vi "Spectrometer.vi"() -> ()   [LabVIEW 2015]
uses:
  <vilib>/Utility/file.llb/Write Delimited Spreadsheet (DBL).vi
panel:
  out "x-y":dbl[](array[numeric])
  out "存储路径":path
  in  "确定按钮":bool
  in  "Stop Spectrum":bool
  out "Backlight Values":dbl[](array[numeric])
  in  "Save Backlight":bool
  in  "Enter the \nInetegration Time":i32=100
  out "Spectrum of the first Spectrometer":cluster{"Y":dbl[], "Y":dbl[]}[](graph)
  in  "Quit Program":bool
  in  "Spectrum Configure":bool
  out "Number of Spectrometers":i32
  # "ms"
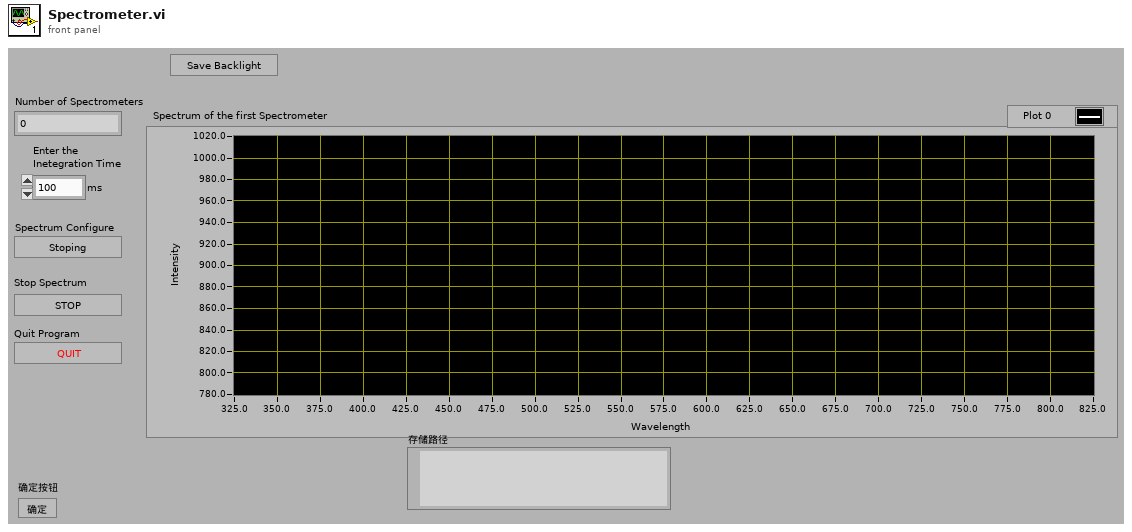
[diagram p1: front panel]
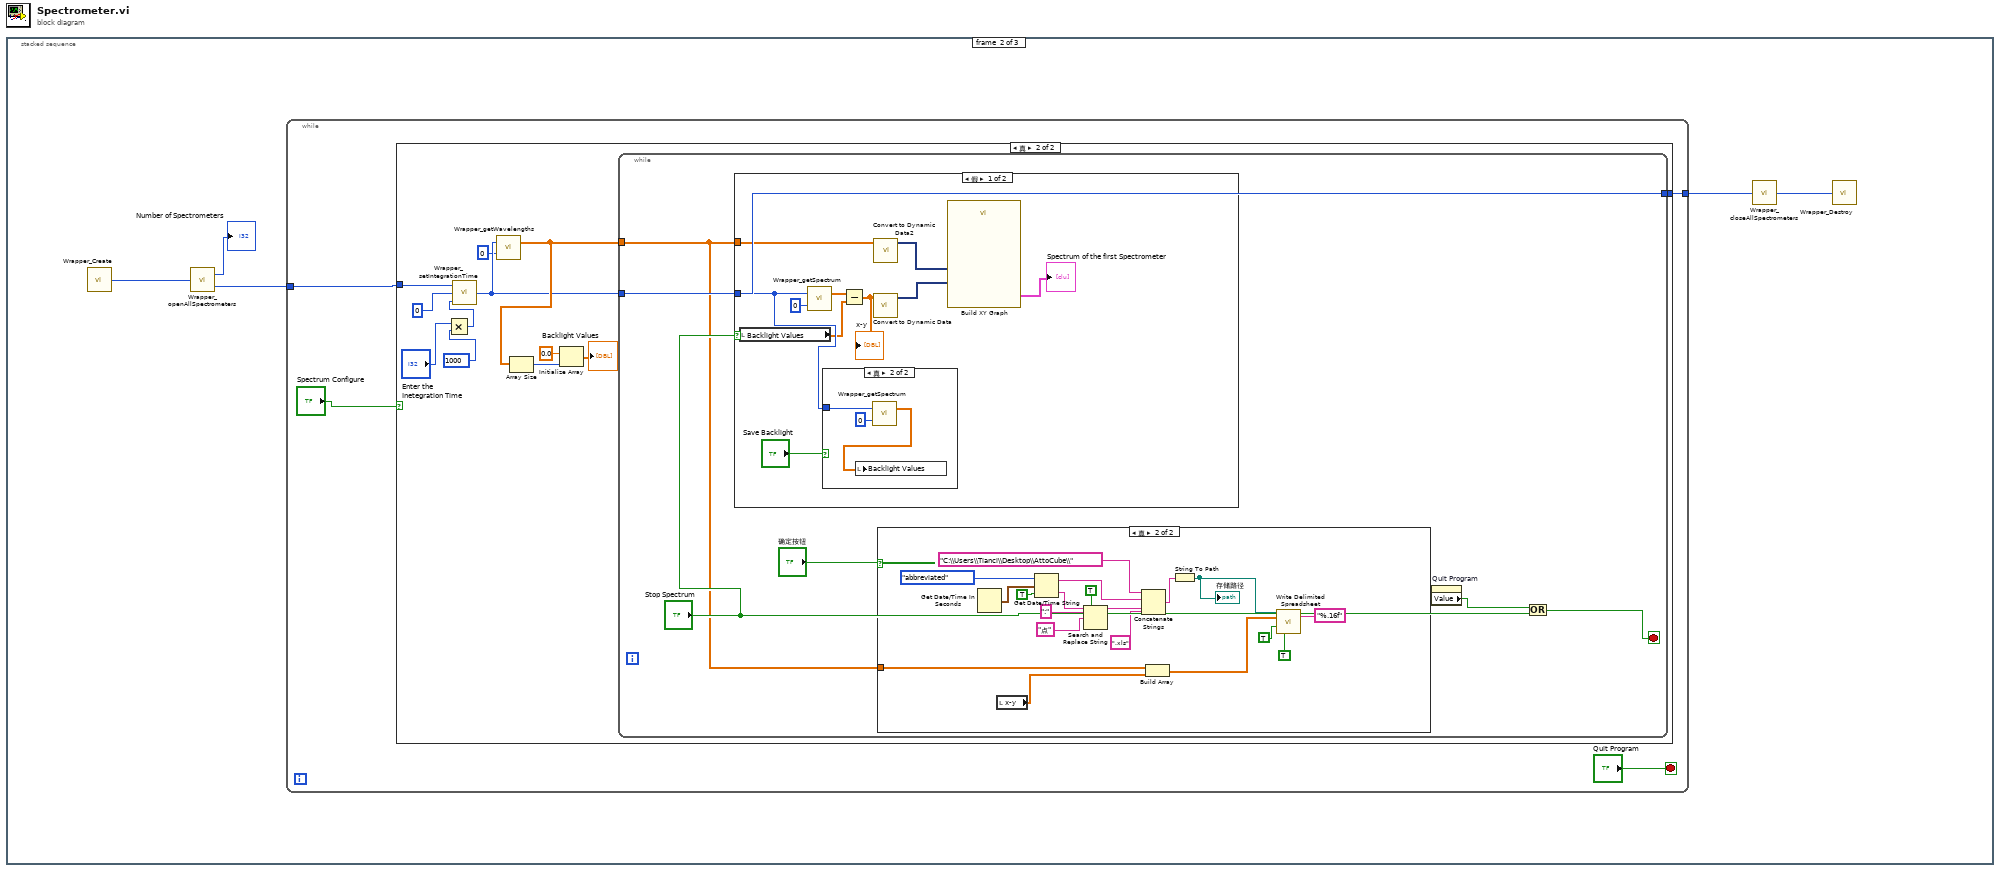
[diagram p0: block diagram]
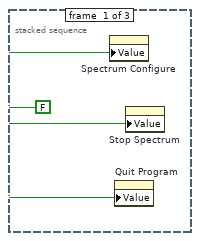
[diagram p2: hidden frame]
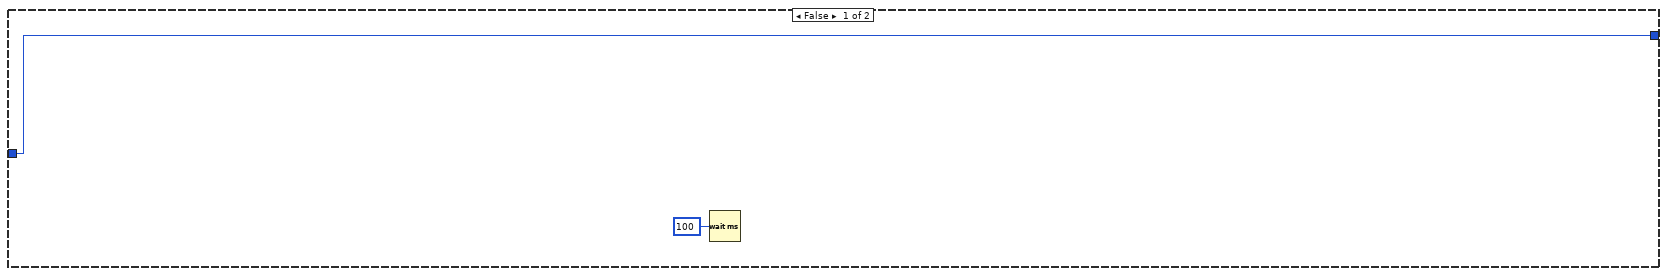
[diagram p3: hidden frame]
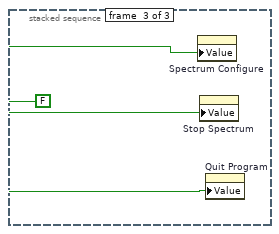
[diagram p7: hidden frame]
diagram:
  n1 = stacked-sequence {
    frame #0 {
      w1 = FALSE
      n2 = property on="Spectrum Configure" class="Bool (严格)"("Value"=w1) -> ()  [unwired: 2 in, 2 out]
      n3 = property on="Quit Program" class="Bool (严格)"("Value"=w1) -> ()  [unwired: 2 in, 2 out]
      n4 = property on="Stop Spectrum" class="Bool (严格)"("Value"=w1) -> ()  [unwired: 2 in, 2 out]
    }
    frame #1 {
      n5 = call <userlib>:"Wrapper_Create.vi"() -> ("Wrapper"=w6:u32)
      n6 = call <userlib>:"Wrapper_openAllSpectrometers.vi"("Wrapper In"=w6) -> ("Number of Spectrometers"=→"Number of Spectrometers":i32, "Wrapper Out"=w5:u32)
      n7 = while {
        tunnel: w5 -> [w10]
        tunnel: [w8] -> w2
        stop <- "Quit Program" stop-if-true
        n8 = case shown="真" "Spectrum Configure" {
          tunnel: w10 -> [w12 w24]
          tunnel: [w12 w21] -> w8
          frame False {
            n9 = Wait (ms)(milliseconds to wait=u32 100 ("等待时间（毫秒）")) -> ()  [unwired: 1 out]
          }
          frame True {
            n10 = Multiply(x="Enter the \nInetegration Time", y=1000) -> (x*y=w13:i32)
            n11 = call <userlib>:"Wrapper_setIntegrationTime.vi"("Integration Time"=w13, "Index"=0, "Wrapper In"=w24) -> ("Wrapper Out"=w22:u32)
            n12 = call <userlib>:"Wrapper_getWavelengths.vi"("Index"=0, "Wrapper"=w22) -> ("WL Values"=w23:dbl[])  [unwired: 1 out]
            n13 = Array Size(array=w23) -> (size(s)=w16:i32)
            n14 = Initialize Array(0.0 ("元素"), w16) -> (→"Backlight Values":dbl[])
            n15 = while {
              tunnel: w23 -> [w25]
              tunnel: w22 -> [w30]
              tunnel: [w30] -> w21
              stop <- w28 stop-if-true
              n16 = case shown="假" "Stop Spectrum" {
                tunnel: w25 -> [w59 _]
                tunnel: w30 -> [w58 _]
                frame False {
                  n17 = local read "Backlight Values"() -> (w50:dbl[])
                  n18 = call <userlib>:"Wrapper_getSpectrum.vi"("Index"=0, "Wrapper"=w58) -> ("Spectrum Values"=w52:dbl[])  [unwired: 1 out]
                  n19 = case shown="真" "Save Backlight" {
                    tunnel: w58 -> [_ w61]
                    frame False {
                    }
                    frame True {
                      n20 = call <userlib>:"Wrapper_getSpectrum.vi"("Index"=0, "Wrapper"=w61) -> ("Spectrum Values"=w60:dbl[])  [unwired: 1 out]
                      n21 = local write "Backlight Values"(w60) -> ()
                    }
                  }
                  n22 = Subtract(x=w52, y=w50) -> (x-y=w51:dbl[])
                  "x-y" <- w51
                  n23 = call "Convert to Dynamic Data"("Array"=w51) -> ("Dynamic Data Type"=w54:dynamicdata)  [unwired: 3 in]
                  n24 = call "Convert to Dynamic Data2"("Array"=w59) -> ("Dynamic Data Type"=w55:dynamicdata)  [unwired: 3 in]
                  n25 = call "Build XY Graph"("Y Input"=w54, "X Input"=w55) -> ("XY Graph"=→"Spectrum of the first Spectrometer":cluster{"Y":dbl[], "Y":dbl[]}[])  [unwired: 8 in, 1 out]
                }
                frame True {
                }
              }
              n26 = case shown="真" "确定按钮" {
                tunnel: w25 -> [_ w33]
                frame False {
                }
                frame True {
                  n27 = Get Date/Time In Seconds() -> (seconds since 1Jan1904=w49:timestamp)
                  n28 = local read "x-y"() -> (w32:dbl[])
                  n29 = Get Date/Time String(date format (0)=enum16{"short", "long", "abbreviated"}."abbreviated" ("日期格式(0)"), seconds (now)=w49, want seconds? (F)=TRUE ("需要秒？(F)")) -> (date string=w41:string, time string=w46:string)
                  n30 = Search and Replace String(replace all?=TRUE ("替换全部？(F)"), input string=w46, search string=":" ("搜索字符串"), replace string="点" ("替换字符串(\"\")")) -> (result string=w42:string)  [unwired: 4 in, 3 out]
                  n31 = Concatenate Strings("C:\\Users\\Tianci\\Desktop\\AttoCube\\" ("字符串"), w41, w42, ".xls" ("字符串")) -> (w40:string)
                  n32 = Build Array(w33, w32) -> (w31:dbl[][])
                  n33 = String To Path(string=w40) -> (path=w37:path)
                  "存储路径" <- w37
                  n34 = call-poly <vilib>:"Write Delimited Spreadsheet.vi"("file path (dialog if empty)"=w37, "format (%.3f)"="%.16f", "2D data"=w31, "append to file? (F)"=TRUE, "transpose? (F)"=TRUE) -> ()  [unwired: 9 in, 2 out]
                }
              }
              n35 = property on="Quit Program" class="Bool (严格)"() -> ("Value"=w29:bool)  [unwired: 2 in, 2 out]
              n36 = Or(x=w29, y="Stop Spectrum") -> (x .or. y?=w28:bool)
            }
          }
        }
      }
      n37 = call <userlib>:"Wrapper_closeAllSpectrometers.vi"("Wrapper In"=w2) -> ("Wrapper Out"=w3:u32)
      n38 = call <userlib>:"Wrapper_Destroy.vi"("Wrapper"=w3) -> ()
    }
    frame #2 {
      w63 = FALSE
      n39 = property on="Spectrum Configure" class="Bool (严格)"("Value"=w63) -> ()  [unwired: 2 in, 2 out]
      n40 = property on="Stop Spectrum" class="Bool (严格)"("Value"=w63) -> ()  [unwired: 2 in, 2 out]
      n41 = property on="Quit Program" class="Bool (严格)"("Value"=w63) -> ()  [unwired: 2 in, 2 out]
    }
  }
